vi "get_depth.vi"(8 "error in (no error)":errorcluster caption="entrée d'erreur (pas d'erreur)", 11 "Tree.lvclass":refnum<class "Tree.lvclass">) -> (0 "error out":errorcluster caption="sortie d'erreur", 2 "depth":i32, 3 "Tree.lvclass 2":refnum<class "Tree.lvclass">)   [LabVIEW 2020, in "Tree.lvclass"]
doc: "Return the depth of the decision tree.\n\nThe depth of a tree is the maximum distance between the root and any leaf."
uses:
  Tree.lvclass
  C:/Users/cipop/TDF Dropbox/2_Technologies de France/1 - Services et Etudes/PLAIY/2 - DEV/PLAIYLAB/code/Python/Python.lvclass
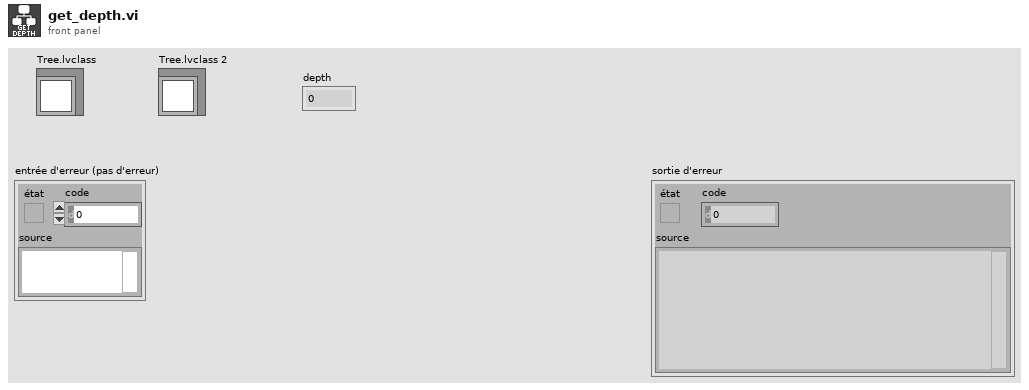
[diagram p1: front panel]
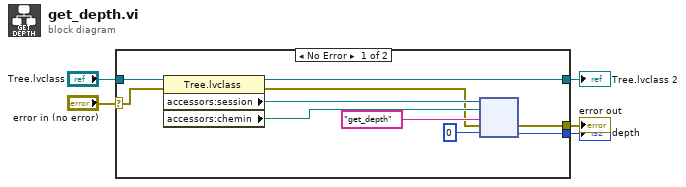
[diagram p0: block diagram]
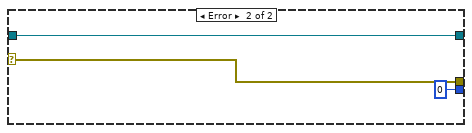
[diagram p2: hidden frame]
diagram:
  n1 = case shown="No Error" "error in (no error)" {
    selector: "error in (no error)" -> [w10 w18]
    tunnel: [w14 w18] -> w4
    tunnel: [w13 w17] -> w2
    tunnel: "Tree.lvclass" -> [w7 w17]
    tunnel: [w6 0] -> w1
    frame No Error {
      n2 = property class="Tree.lvclass"(reference=w7, error in=w10) -> (reference out=w13:refnum<class "Tree.lvclass">, error out=w9:errorcluster, "accessors:session"=w12:refnum<k35>, "accessors:chemin"=w11:path)
      n3 = node(w12, w11, "get_depth" ("nom de la fonction"), w9, 0) -> (w14:errorcluster, w6:i32)  [unwired: 3 out]
    }
    frame Error {
    }
  }
  "error out" <- w4
  "Tree.lvclass 2" <- w2
  "depth" <- w1
